vi "DE_PARTICLE_REPORT_TO_ORDER(SubVI).vi"(3 "put in order":u16(ring) items=["Max. Area", "Min. Area", "Max. Center of Mass", "Min. Center of Mass"], 4 "Particle Reports (Pixels)":T1(array[cluster]) {"Orientation" format="%.2f"; "Dimensions"."Height" format="%.2f"; "Dimensions"."Width" format="%.2f"; "Center of Mass"."Y" format="%.2f"; "Center of Mass"."X" format="%.2f"; "Bounding Rect"."Bottom" format="%.2f"; "Bounding Rect"."Right" format="%.2f"; "Bounding Rect"."Top" format="%.2f"; "Bounding Rect"."Left" format="%.2f"; "Number of Holes" format="%.2f"; "Area" format="%.2f"}) -> (1 "Particle Reports (Pixels) 2":T1(array[cluster]) {"Orientation" format="%.2f"; "Dimensions"."Height" format="%.2f"; "Dimensions"."Width" format="%.2f"; "Center of Mass"."Y" format="%.2f"; "Center of Mass"."X" format="%.2f"; "Bounding Rect"."Bottom" format="%.2f"; "Bounding Rect"."Right" format="%.2f"; "Bounding Rect"."Top" format="%.2f"; "Bounding Rect"."Left" format="%.2f"; "Number of Holes" format="%.2f"; "Area" format="%.2f"})   [LabVIEW 2011]
doc: "Ordena los resultados del shape match tool a max. o min. object size y max. o . min score."
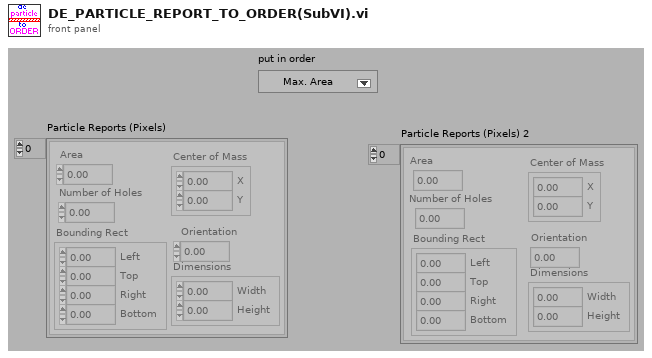
[diagram p1: front panel]
types:
  T1 = cluster{"Area":dbl, "Number of Holes":dbl, "Bounding Rect":cluster{"Left":dbl, "Top":dbl, "Right":dbl, "Bottom":dbl}, "Center of Mass":cluster{"X":dbl, "Y":dbl}, "Orientation":dbl, "Dimensions":cluster{"Width":dbl, "Height":dbl}}[]
  T2 = cluster{"Area":dbl, "Number of Holes":dbl, "Bounding Rect":cluster{"Left":dbl, "Top":dbl, "Right":dbl, "Bottom":dbl}, "Center of Mass":cluster{"X":dbl, "Y":dbl}, "Orientation":dbl, "Dimensions":cluster{"Width":dbl, "Height":dbl}}
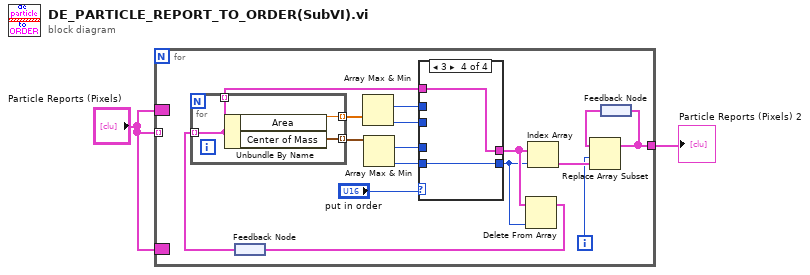
[diagram p0: block diagram]
diagram:
  n1 = for {
    tunnel: "Particle Reports (Pixels)" -> [_] mode=indexing
    tunnel: [w3] -> w1
    border: "Particle Reports (Pixels)" -> [_]
    border: "Particle Reports (Pixels)" -> [_]
    i -> [w5]
    n2 = feedback #1() -> (w8:T1)
    n3 = for {
      tunnel: w8 -> [w27] mode=indexing
      tunnel: [w29] -> w18 mode=indexing
      tunnel: [w28] -> w17 mode=indexing
      tunnel: [w27] -> w15 mode=indexing
      n4 = Unbundle By Name(w27) -> ("Area"=w29:dbl, "Center of Mass"=w28:cluster{"X":dbl, "Y":dbl})
    }
    n5 = Array Max & Min(array=w18) -> (max index (indices)=w16:i32, min index (indices)=w13:i32)  [unwired: 2 out]
    n6 = Array Max & Min(array=w17) -> (max index (indices)=w12:i32, min index (indices)=w11:i32)  [unwired: 2 out]
    n7 = case shown="3" "put in order" {
      tunnel: w15 -> [w19 w22 w24 w26]
      tunnel: w16 -> [w20 _ _ _]
      tunnel: [w19 w22 w24 w26] -> w10
      tunnel: [w20 w21 w23 w25] -> w9
      tunnel: w13 -> [_ w21 _ _]
      tunnel: w12 -> [_ _ w23 _]
      tunnel: w11 -> [_ _ _ w25]
      frame 0, Default {
      }
      frame 1 {
      }
      frame 2 {
      }
      frame 3 {
      }
    }
    n8 = Delete From Array(array=w10, index=w9) -> (array with subset deleted=w7:T1)  [unwired: 1 in, 1 out]
    n9 = feedback-in #1(w7) -> ()
    n10 = Index Array(array=w10, index=w9) -> (element=w6:T2)
    n11 = feedback #2() -> (w4:T1)
    n12 = Replace Array Subset(array=w4, new element=w6, index=w5) -> (w3:T1)
    n13 = feedback-in #2(w3) -> ()
  }
  "Particle Reports (Pixels) 2" <- w1
